vi "checkout.vi"(7 "locked by?":string, 8 "error in (no error)":errorcluster) -> (0 "error out":errorcluster, 3 "GenericStage out":refnum<class "GenericStage.lvclass">)   [LabVIEW 2010, in "GenericStage.lvclass"]
uses:
  GenericStage.lvclass
  class_data.vi
  common/classes/ErrorController/ErrorController/class_data.vi
  common/classes/GenericComponent/GenericComponent/GenericComponent.lvclass
  common/classes/ErrorController/ErrorController/ErrorController.lvclass
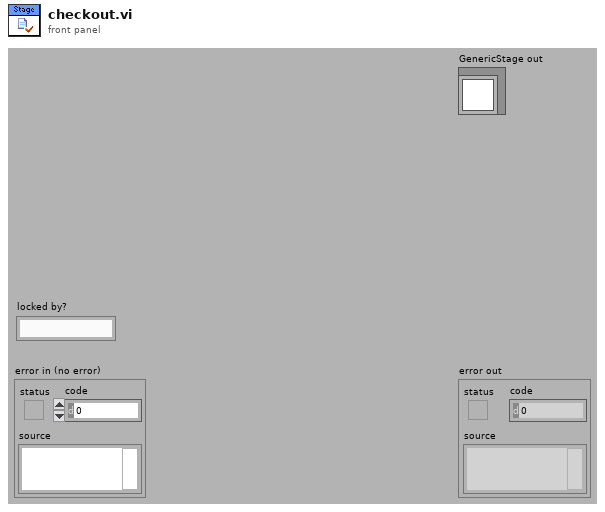
[diagram p1: front panel]
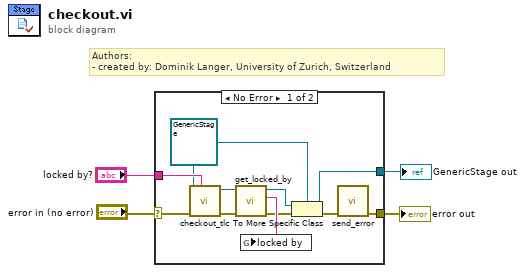
[diagram p0: block diagram]
diagram:
  # "Authors: \n- created by: Dominik Langer, University of Zurich, Switzerland"
  n1 = case shown="No Error" "error in (no error)" {
    selector: "error in (no error)" -> [w8 w16]
    tunnel: [w6 w16] -> w3
    tunnel: [w10 _] -> w2
    tunnel: "locked by?" -> [w9 _]
    frame No Error {
      w5 = refnum<class "GenericStage.lvclass"> refnum ("GenericStage.lvclass")
      n2 = call-dynamic "checkout_tlc.vi"("locked by?"=w9, "error in (no error)"=w8, "GenericToplevelComponent in"=w5) -> ("error out"=w14:errorcluster, "GenericToplevelComponent out"=w15:refnum<class "GenericToplevelComponent.lvclass">)  [unwired: 7 in]
      n3 = call "get_locked_by.vi"("error in (no error)"=w14, "GenericPlugin.lvclass in"=w15) -> ("error out"=w11:errorcluster, "locked by"=w13:string, "GenericPlugin.lvclass out"=w12:refnum<class "GenericToplevelComponent.lvclass">)  [unwired: 7 out]
      n4 = global write "class_data.vi" "locked by"(w13) -> ()
      n5 = To More Specific Class(target class=w5, reference=w12, error in=w11) -> (specific class reference=w10:refnum<class "GenericStage.lvclass">, error out=w7:errorcluster)
      n6 = call "send_error.vi"("error in (no error)"=w7) -> ("error out"=w6:errorcluster)  [unwired: 10 in]
    }
    frame Error {
    }
  }
  "error out" <- w3
  "GenericStage out" <- w2
